vi "Select_events.vi"(8 "error in (no error)":errorcluster, 9 "Select errored events":bool, 10 "Small?":bool, 11 "Constraints":T1 {"Estimate Quality" scale=0.0..5.0; "Lower Mass Limit (kg)" min=-1.0 max=1.0 step=1e-20; "Upper Mass Limit (kg)" min=-1.0 max=1.0 step=1e-20; "Lower Velocity Limit (km/s)" min=-1.0 max=299792000.0; "Upper Velocity Limit (km/s)" min=-1.0 max=299792000.0}) -> (0 "error out":errorcluster, 3 "Dust Events":i64[](array[numeric]))   [LabVIEW 2013]
uses:
  Controls/Constraints.ctl
  <vilib>/addons/database/Auxilliary.llb/DB Tools Cursor Type.ctl
  <userlib>/_OpenG.lib/array/array.llb/Remove Duplicates from 1D Array (String)__ogtk.vi
  <userlib>/_OpenG.lib/array/array.llb/Search 1D Array (String)__ogtk.vi
  <userlib>/_OpenG.lib/array/array.llb/Delete Elements from 1D Array (String)__ogtk.vi
  <vilib>/addons/database/Connection.llb/Conn Execute.vi
  <vilib>/addons/database/Recordset.llb/Rec Fetch Recordset Data (R).vi
  <vilib>/addons/database/Recordset.llb/Rec Destroy - Connection.vi
  <vilib>/addons/database/_DB Variant To Data/Database Variant To Data.xnode
  <vilib>/addons/database/NI_Database_API.lvlib
panel:
  out "Select Events Syntax":string
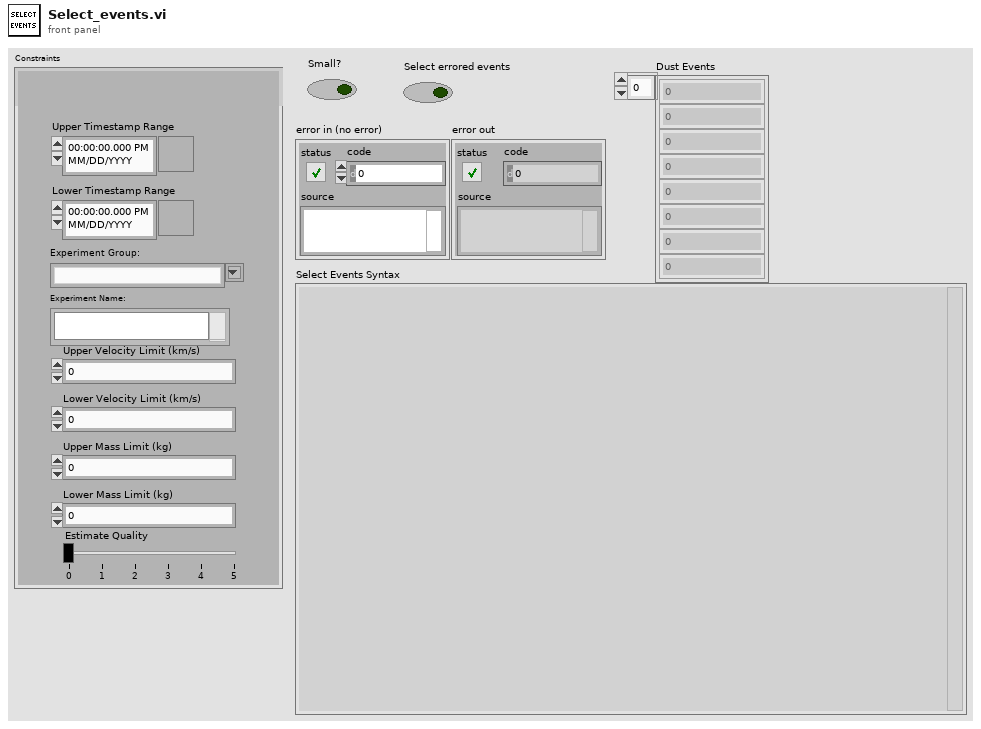
[diagram p1: front panel]
types:
  T1 = typedef "Constraints.ctl" = cluster{"Upper Timestamp Range":timestamp, "Lower Timestamp Range":timestamp, "Experiment Group:":string, "Experiment Name:":i32[], "Upper Velocity Limit (km/s)":dbl, "Lower Velocity Limit (km/s)":dbl, "Upper Mass Limit (kg)":dbl, "Lower Mass Limit (kg)":dbl, "name array":string[], "Estimate Quality":cluster{dbl, dbl}}
  T2 = typedef "NI_Database_API.lvlib/DB Tools Cursor Type.ctl" = enum16{"forward-only", "keyset", "dynamic", "static"}
  T3 = typedef "NI_Database_API.lvlib/Conn ObjectReference.ctl" = refnum<k1>
  T4 = typedef "NI_Database_API.lvlib/Rec ObjectReference.ctl" = refnum<k1>
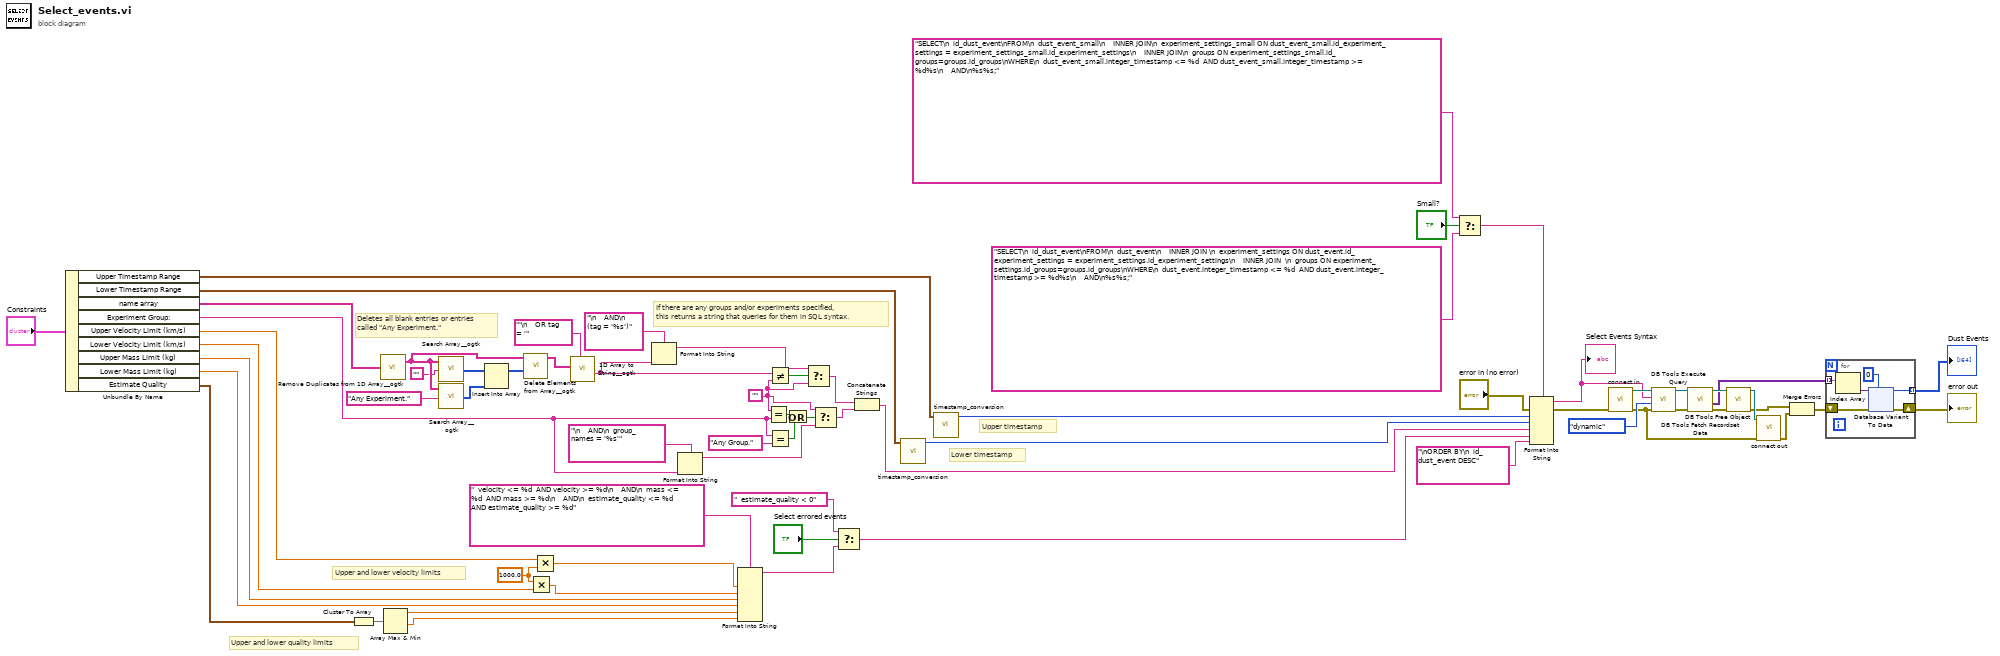
[diagram p0: block diagram]
diagram:
  w3 = ""
  w43 = 1000.0 ("y")
  # "Upper and lower velocity limits"
  # "Deletes all blank entries or entries\ncalled \"Any Experiment.\""
  # "Upper and lower quality limits"
  # "Lower timestamp"
  # "Upper timestamp"
  # "If there are any groups and/or experiments specified,\nthis returns a string that queries for them in SQL syntax."
  n1 = Unbundle By Name("Constraints") -> ("Upper Timestamp Range"=w23:timestamp, "Lower Timestamp Range"=w22:timestamp, "name array"=w19:string[], "Experiment Group:"=w2:string, "Upper Velocity Limit (km/s)"=w13:dbl, "Lower Velocity Limit (km/s)"=w12:dbl, "Upper Mass Limit (kg)"=w9:dbl, "Lower Mass Limit (kg)"=w8:dbl, "Estimate Quality"=w36:cluster{dbl, dbl})
  n2 = Cluster To Array(cluster=w36) -> (array=w44:dbl[])
  n3 = call-poly <userlib>:"Remove Duplicates from 1D Array__ogtk.vi"("Input Array"=w19) -> ("Output Array"=w63:string[])  [unwired: 1 out]
  n4 = Array Max & Min(array=w44) -> (max value=w7:dbl, min value=w6:dbl)  [unwired: 2 out]
  n5 = call-poly <userlib>:"Search Array__ogtk.vi"("Array"=w63, "Element Data"="") -> ("Indices of Elements"=w47:i32[])  [unwired: 7 in]
  n6 = call-poly <userlib>:"Search Array__ogtk.vi"("Array"=w63, "Element Data"="Any Experiment.") -> ("Indices of Elements"=w65:i32[])  [unwired: 7 in]
  n7 = Insert Into Array(array=w47, new element=w65) -> (w64:i32[])  [unwired: 1 in]
  n8 = call-poly <userlib>:"Delete Elements from Array__ogtk.vi"("indices"=w64, "array"=w63) -> ("array w/ subset deleted"=w18:string[])  [unwired: 8 in, 1 out]
  n9 = Multiply(x=w43, y=w12) -> (x*y=w10:dbl)
  n10 = Multiply(x=w13, y=w43) -> (x*y=w11:dbl)
  n11 = call <userlib>:"1D Array to String__ogtk.vi"("delimiter (Tab)"="'\n    OR tag = '", "Array of Strings"=w18) -> ("delimited string"=w51:string)  [unwired: 9 in]
  n12 = Format Into String(format string="\n    AND\n  (tag = '%s')" ("string"), w51) -> (resulting string=w67:string)  [unwired: 2 in, 1 out]
  n13 = Format Into String(format string="\n    AND\n  group_names = '%s'" ("string"), w2) -> (resulting string=w41:string)  [unwired: 2 in, 1 out]
  n14 = Format Into String(format string="  velocity <= %d  AND velocity >= %d\n    AND\n  mass <= %d  AND mass >= %d\n    AND\n  estimate_quality <= %d AND estimate_quality >= %d" ("input 10"), w11, w10, w9, w8, w7, w6) -> (resulting string=w16:string)  [unwired: 2 in, 1 out]
  n15 = Equal?(x=w3, y=w2) -> (x = y?=w50:bool)
  n16 = Not Equal?(x=w51, y=w3) -> (x != y?=w66:bool)
  n17 = Equal?(x=w2, y="Any Group.") -> (x = y?=w48:bool)
  n18 = Or(x=w50, y=w48) -> (x .or. y?=w49:bool)
  n19 = Select(t=w67, s=w66, f=w3) -> (s? t:f=w38:string)
  n20 = Select(t=w3, s=w49, f=w41) -> (s? t:f=w39:string)
  n21 = Select(t="  estimate_quality < 0", s="Select errored events", f=w16) -> (s? t:f=w5:string)
  n22 = Concatenate Strings(w38, w39) -> (w61:string)
  n23 = call "timestamp_conversion.vi"("Time Stamp"=w22) -> ("Integer Time"=w60:i64)  [unwired: 8 in, 1 out]
  n24 = call "timestamp_conversion.vi"("Time Stamp"=w23) -> ("Integer Time"=w59:i64)  [unwired: 8 in, 1 out]
  n25 = Select(t="SELECT\n  id_dust_event\nFROM\n  dust_event_small\n    INNER JOIN\n  experiment_settings_small ON dust_event_small.id_experiment_settings = experiment_settings_small.id_experiment_settings\n    INNER JOIN\n  groups ON experiment_settings_small.id_groups=groups.id_groups\nWHERE\n  dust_event_small.integer_timestamp <= %d  AND dust_event_small.integer_timestamp >= %d%s\n    AND\n%s%s;" ("string"), s="Small?", f="SELECT\n  id_dust_event\nFROM\n  dust_event\n    INNER JOIN \n  experiment_settings ON dust_event.id_experiment_settings = experiment_settings.id_experiment_settings\n    INNER JOIN  \n  groups ON experiment_settings.id_groups=groups.id_groups\nWHERE\n  dust_event.integer_timestamp <= %d  AND dust_event.integer_timestamp >= %d%s\n    AND\n%s%s;" ("string")) -> (s? t:f=w25:string)
  n26 = Format Into String(format string=w25, error in="error in (no error)", w59, w60, w61, w5, "\nORDER BY\n  id_dust_event DESC" ("input 5")) -> (resulting string=w24:string, error out=w54:errorcluster)  [unwired: 1 in]
  "Select Events Syntax" <- w24
  n27 = call "connect in.vi"("error in (no error)"=w54) -> ("error out"=w31:errorcluster, "Database Connection"=w55:T3)  [unwired: 6 in, 1 out]
  n28 = call-poly <vilib>:"DB Tools Execute Query.vi"("error in (no error)"=w31, "cursor type"=DB_Tools_Cursor_Type."dynamic", "SQL query"=w24, "connection reference"=w55) -> ("error out"=w58:errorcluster, "recordset reference"=w57:T4)  [unwired: 4 in]
  n29 = call-poly <vilib>:"DB Tools Fetch Recordset Data.vi"("error in (no error)"=w58, "recordset reference"=w57) -> ("error out"=w53:errorcluster, "recordset data"=w21:variant[][], "recordset reference out"=w56:T4)  [unwired: 3 in]
  n30 = call-poly <vilib>:"DB Tools Free Object.vi"("error in (no error)"=w53, "recordset reference"=w56) -> ("error out"=w34:errorcluster, "connection reference"=w35:T3)  [unwired: 8 in]
  n31 = call "connect out.vi"("error in (no error)"=w31, "connection reference"=w35) -> ("error out"=w33:errorcluster)  [unwired: 9 in]
  n32 = Merge Errors(w34, w33) -> (w32:errorcluster)
  n33 = for {
    tunnel: [w71] -> w20 mode=indexing
    tunnel: w21 -> [w68] mode=indexing
    shift-right: [w72] -> w29
    shift-left: w32 -> [w73]
    n34 = Index Array(array=w68) -> (element=w70:variant)  [unwired: 1 in]
    n35 = xnode "Database Variant To Data"("database variant"=w70, "error in (no error)"=w73, "type"=i64 0 ("Number of Events")) -> ("data"=w71:i64, "error out"=w72:errorcluster)
  }
  "error out" <- w29
  "Dust Events" <- w20
